vi "FindClassObject.vi"(1 "full class name":string, 5 "error in (no error)":errorcluster) -> (14 "proxy class object ref":refnum<class "G#RemoteProxy.lvclass">, 15 "not found?":bool, 19 "error out":errorcluster)   [LabVIEW 2017, in "G#RemoteProxy.lvclass"]
doc: "Finds the class object specified by the full class name."
uses:
  <vilib>/addons/_AddQ/G#Debugger/G#RemoteProxy/G#RemoteProxy.lvclass
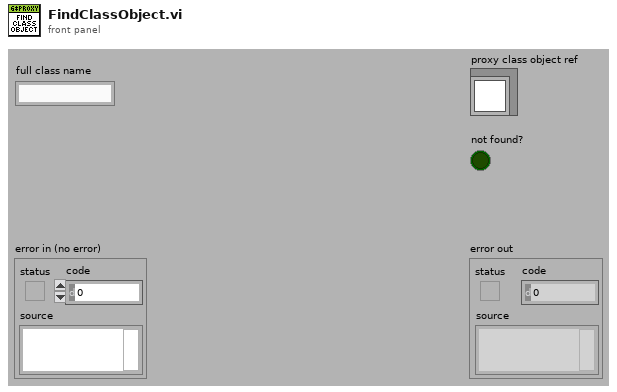
[diagram p1: front panel]
types:
  T1 = typedef "G#RemoteProxy.lvclass/ClassAttributesRef.ctl" = refnum<data-value>
  T2 = typedef "G#RemoteProxy.lvclass/ClassAttributesProxy.ctl" = cluster{"NoActiveProject":bool, "FullClassNames":string[], "FullClassPaths":path[], "RemoteRefs":refnum<class "G#Object.lvclass">[], "ProxyRefs":refnum<class "G#RemoteProxy.lvclass">[], "RemoteClassName":string[], "ProxyClassRefs":refnum<class "G#RemoteProxy.lvclass">[]}
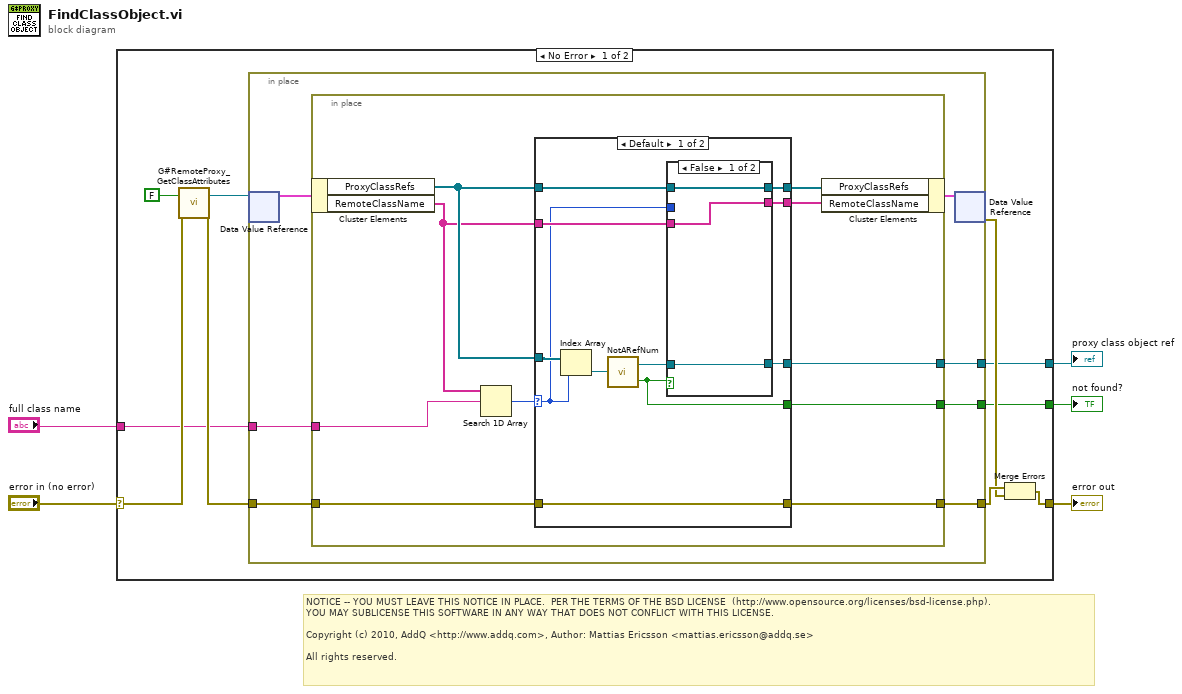
[diagram p0: block diagram]
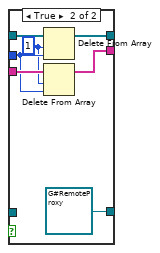
[diagram p2: hidden frame]
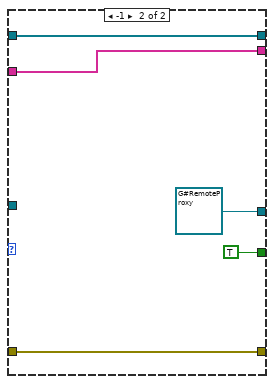
[diagram p3: hidden frame]
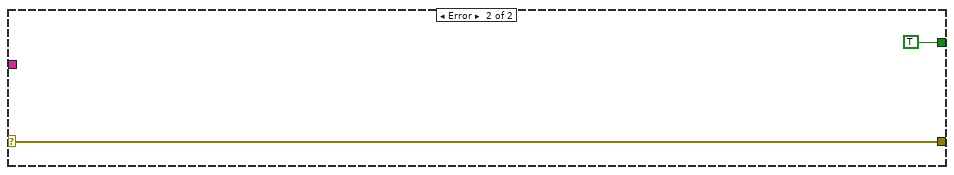
[diagram p4: hidden frame]
diagram:
  # "NOTICE -- YOU MUST LEAVE THIS NOTICE IN PLACE.  PER THE TERMS OF THE BSD LICENSE  (http://www.opensource.org/licenses/bsd-license.php).\nYOU MAY SUBLICENSE THIS SOFTWARE IN ANY WAY THAT DOES NOT CONFLICT WITH THIS LICENSE.\n\nCopyright (c) 2010, AddQ <http://www.addq.com>, Author: Mattias Ericsson <mattias.ericsson@addq.se>\n\nAll rights reserved."
  n1 = case shown="No Error" "error in (no error)" {
    selector: "error in (no error)" -> [w15 w60]
    tunnel: [w12 w60] -> w4
    tunnel: "full class name" -> [w8 _]
    tunnel: [w7 _] -> w2
    tunnel: [w6 TRUE ("not a refnum?")] -> w1
    frame No Error {
      n2 = call <vilib>:"G#RemoteProxy_GetClassAttributes.vi"("return data? (T)"=FALSE ("return data"), "error in (no error)"=w15) -> ("class attributes ref"=w13:T1, "error out"=w14:errorcluster)  [unwired: 14 in, 2 out]
      n3 = in-place {
        in-place-border: w14 -> [w19]
        in-place-border: [w18] -> w10
        in-place-border: w8 -> [w20]
        in-place-border: [w17] -> w7
        in-place-border: [w16] -> w6
        n4 = in-place-dvr #1(w13) -> (w21:T2)  [unwired: 1 out]
        n5 = in-place {
          in-place-border: w20 -> [w29]
          in-place-border: w19 -> [w31]
          in-place-border: [w30] -> w18
          in-place-border: [w28] -> w17
          in-place-border: [w27] -> w16
          n6 = in-place-cluster #2(w21) -> ("ProxyClassRefs"=w26:refnum<class "G#RemoteProxy.lvclass">[], "RemoteClassName"=w24:string[])
          n7 = Search 1D Array(1D array=w24, element=w29) -> (index of element=w32:i32)  [unwired: 1 in]
          n8 = case shown="Default" w32 {
            selector: w32 -> [w35 _]
            tunnel: w31 -> [w43 w58]
            tunnel: [w43 w58] -> w30
            tunnel: w26 -> [w42 _]
            tunnel: [w40 refnum<class "G#RemoteProxy.lvclass"> refnum ("ProxyClassObject")] -> w28
            tunnel: [w34 TRUE] -> w27
            tunnel: w26 -> [w39 w55]
            tunnel: [w38 w55] -> w25
            tunnel: w24 -> [w37 w54]
            tunnel: [w36 w54] -> w23
            frame Default {
              n9 = Index Array(array=w42, index=w35) -> (element=w41:refnum<class "G#RemoteProxy.lvclass">)
              n10 = call-dynamic "NotARefNum.vi"("reference in"=w41) -> ("not a refnum?"=w34:bool, "reference out"=w33:refnum<class "G#RemoteProxy.lvclass">)  [unwired: 1 in]
              n11 = case shown="False" w34 {
                tunnel: [w44 refnum<class "G#RemoteProxy.lvclass"> refnum ("ProxyClassObject")] -> w40
                tunnel: w39 -> [w46 w52]
                tunnel: [w46 w51] -> w38
                tunnel: w37 -> [w45 w50]
                tunnel: [w45 w49] -> w36
                tunnel: w35 -> [_ w48]
                tunnel: w33 -> [w44 _]
                frame False {
                }
                frame True {
                  w47 = 1 ("length")
                  n12 = Delete From Array(array=w52, length=w47, index=w48) -> (array with subset deleted=w51:refnum<class "G#RemoteProxy.lvclass">[])  [unwired: 1 out]
                  n13 = Delete From Array(array=w50, length=w47, index=w48) -> (array with subset deleted=w49:string[])  [unwired: 1 out]
                }
              }
            }
            frame -1 {
            }
          }
          n14 = in-place-cluster #2("ProxyClassRefs"=w25, "RemoteClassName"=w23) -> (w22:T2)
        }
        n15 = in-place-dvr #1(w22) -> (w9:errorcluster)  [unwired: 1 out]
      }
      n16 = Merge Errors(w10, w9) -> (w12:errorcluster)
    }
    frame Error {
    }
  }
  "error out" <- w4
  "proxy class object ref" <- w2
  "not found?" <- w1
